vi "app_runner.vi"() -> ()   [LabVIEW 2020]
uses:
  #typedefs/#typedef_enum_QueueActions.ctl
panel:
  in  "Play Button":bool
  # "Image Analyzer App"
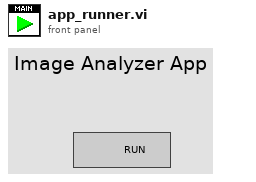
[diagram p1: front panel]
types:
  T1 = typedef "#typedef_enum_QueueActions.ctl" = enum16{"Obtain", "GetRef", "Enqueue", "Release"}
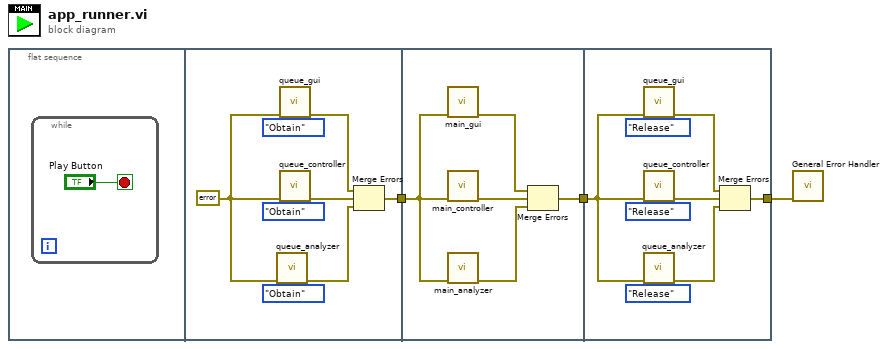
[diagram p0: block diagram]
diagram:
  n1 = flat-sequence {
    tunnel: [w8] -> w3
    tunnel: w3 -> [w14]
    tunnel: [w15] -> w2
    tunnel: w2 -> [w19]
    tunnel: [w21] -> w1
    frame #0 {
      n2 = while {
        stop <- "Play Button" stop-if-true
      }
    }
    frame #1 {
      w6 = errorcluster {"status"=FALSE, "code"=0, "source"=""} ("error constant")
      n3 = call "queue_analyzer.vi"("QueueActions"=#typedef_enum_QueueActions."Obtain", "error in (no error)"=w6) -> ("error out"=w5:errorcluster)  [unwired: 8 in, 1 out]
      n4 = call "queue_gui.vi"("QueueActions"=#typedef_enum_QueueActions."Obtain", "error in (no error)"=w6) -> ("error out"=w10:errorcluster)  [unwired: 8 in, 1 out]
      n5 = call "queue_controller.vi"("QueueActions"=#typedef_enum_QueueActions."Obtain", "error in (no error)"=w6) -> ("error out"=w9:errorcluster)  [unwired: 8 in, 1 out]
      n6 = Merge Errors(w10, w9, w5) -> (w8:errorcluster)
    }
    frame #2 {
      n7 = call "main_gui.vi"("error in (no error)"=w14) -> ("error out"=w16:errorcluster)  [unwired: 10 in]
      n8 = call "main_controller.vi"("error in"=w14) -> ("error out"=w17:errorcluster)  [unwired: 10 in]
      n9 = call "main_analyzer.vi"("error in (no error)"=w14) -> ("error out"=w13:errorcluster)  [unwired: 10 in]
      n10 = Merge Errors(w16, w17, w13) -> (w15:errorcluster)
    }
    frame #3 {
      n11 = call "queue_gui.vi"("QueueActions"=#typedef_enum_QueueActions."Release", "error in (no error)"=w19) -> ("error out"=w23:errorcluster)  [unwired: 8 in, 1 out]
      n12 = call "queue_controller.vi"("QueueActions"=#typedef_enum_QueueActions."Release", "error in (no error)"=w19) -> ("error out"=w22:errorcluster)  [unwired: 8 in, 1 out]
      n13 = call "queue_analyzer.vi"("QueueActions"=#typedef_enum_QueueActions."Release", "error in (no error)"=w19) -> ("error out"=w18:errorcluster)  [unwired: 8 in, 1 out]
      n14 = Merge Errors(w23, w22, w18) -> (w21:errorcluster)
    }
  }
  n15 = call <vilib>:"General Error Handler.vi"("error in (no error)"=w1) -> ()  [unwired: 10 in, 5 out]
